vi "Configure Harmonic.vi"(0 "VISA resource name":refnum<visa-resource-name>, 1 "Serial Number (2)":i32=2, 2 "Phase (0 Degree)":i32, 5 "Output Channel (1: Channel 1)":i32(ring)=1 items=["Channel 1"=1, "Channel 2"=2], 7 "Order (2)":i32=2, 9 "Harmonic Type (0: Even)":i32(ring) items=["Even", "Odd", "All", "User"], 11 "error in (no error)":errorcluster, 12 "Amplitude (1.2647 Vpp)":dbl=1.2647) -> (4 "VISA resource name out":refnum<visa-resource-name>, 15 "error out":errorcluster)   [LabVIEW 2015, in "RIGOL DG4000 Series.lvlib"]
doc: "Configures the harmonic order, harmonic type, the amplitude and phase of specified order of harmonic."
uses:
  <instrlib>/RIGOL DG4000 Series/RIGOL DG4000 Series.lvlib
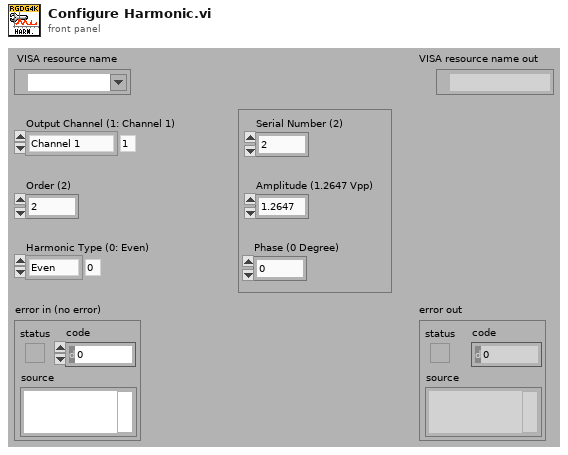
[diagram p1: front panel]
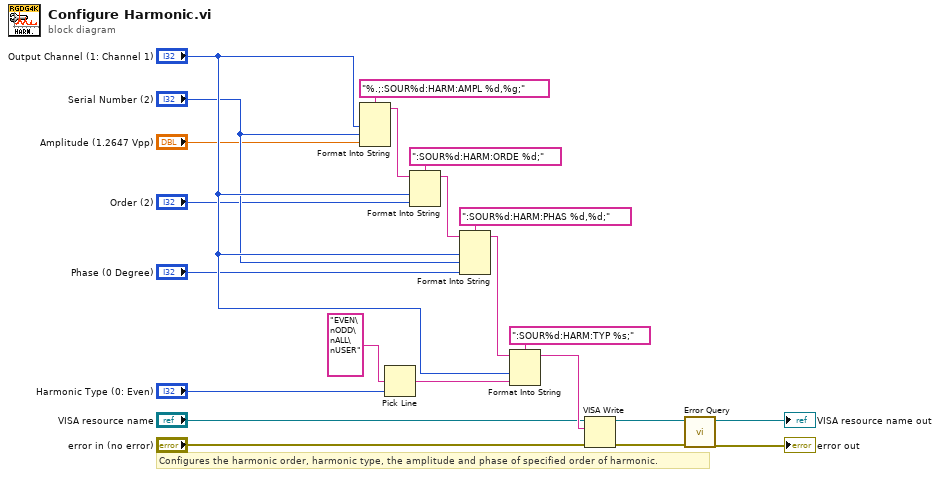
[diagram p0: block diagram]
diagram:
  # "Configures the harmonic order, harmonic type, the amplitude and phase of specified order of harmonic."
  n1 = Format Into String(format string="%.;:SOUR%d:HARM:AMPL %d,%g;", "Output Channel (1: Channel 1)", "Serial Number (2)", "Amplitude (1.2647 Vpp)") -> (resulting string=w18:string)  [unwired: 2 in, 1 out]
  n2 = Pick Line(multi-line string="EVEN\nODD\nALL\nUSER", line index="Harmonic Type (0: Even)") -> (output string=w8:string)  [unwired: 1 out]
  n3 = Format Into String(format string=":SOUR%d:HARM:ORDE %d;", initial string=w18, "Output Channel (1: Channel 1)", "Order (2)") -> (resulting string=w15:string)  [unwired: 1 in, 1 out]
  n4 = Format Into String(format string=":SOUR%d:HARM:PHAS %d,%d;", initial string=w15, "Output Channel (1: Channel 1)", "Serial Number (2)", "Phase (0 Degree)") -> (resulting string=w10:string)  [unwired: 1 in, 1 out]
  n5 = Format Into String(format string=":SOUR%d:HARM:TYP %s;", initial string=w10, "Output Channel (1: Channel 1)", w8) -> (resulting string=w7:string)  [unwired: 1 in, 1 out]
  n6 = VISA Write(VISA resource name="VISA resource name", write buffer=w7, error in (no error)="error in (no error)") -> (VISA resource name out=w4:refnum<visa-resource-name>, error out=w3:errorcluster)  [unwired: 1 out]
  n7 = call <instrlib>:"Error Query.vi"("error in (no error)"=w3, "VISA resource name"=w4) -> ("error out"=→"error out":errorcluster, "VISA resource name out"=→"VISA resource name out":refnum<visa-resource-name>)  [unwired: 8 out]
